vi "Wait for application to close.vi"(8 "error in (no error)":errorcluster, 11 "Applcation name":string="C:\\\\WINDOWS\\\\SYSTEM32\\\\cmd.exe") -> (0 "error out":errorcluster)   [LabVIEW 2013]
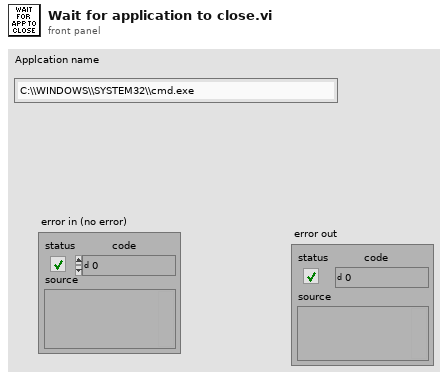
[diagram p1: front panel]
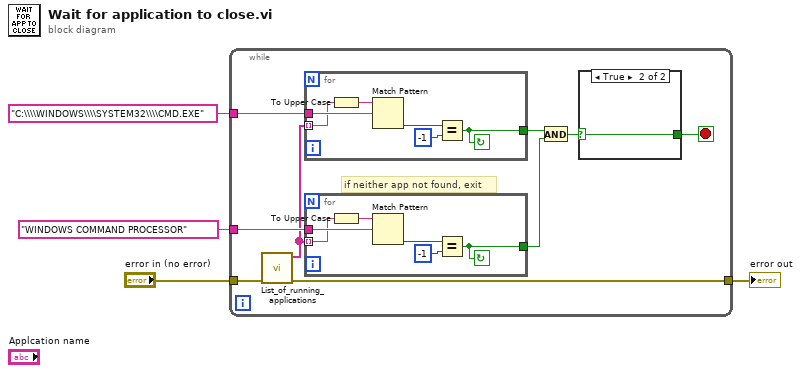
[diagram p0: block diagram]
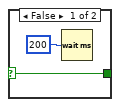
[diagram p2: hidden frame]
diagram:
  n1 = while {
    tunnel: "error in (no error)" -> [w12]
    tunnel: [w11] -> w3
    tunnel: "WINDOWS COMMAND PROCESSOR" -> [w10]
    tunnel: "C:\\\\WINDOWS\\\\SYSTEM32\\\\CMD.EXE" ("Applcation name") -> [w8]
    stop <- w13 stop-if-true
    # "if neither app not found, exit"
    n2 = call "List_of_running_applications.vi"("error in (no error)"=w12) -> ("error out"=w11:errorcluster, "TaskManager's list"=w9:string[])  [unwired: 7 in]
    n3 = for {
      tunnel: w9 -> [w15] mode=indexing
      tunnel: [w16] -> w7
      tunnel: w8 -> [w17]
      stop <- w16 continue-if-true
      n4 = To Upper Case(1:w15) -> (0:w14:string)
      n5 = Match Pattern(string=w14, regular expression=w17) -> (offset past match=w19:i32)  [unwired: 1 in, 3 out]
      n6 = Equal?(x=w19, y=-1) -> (x = y?=w16:bool)
    }
    n7 = for {
      tunnel: w9 -> [w24] mode=indexing
      tunnel: [w26] -> w6
      tunnel: w10 -> [w25]
      stop <- w26 continue-if-true
      n8 = To Upper Case(1:w24) -> (0:w23:string)
      n9 = Match Pattern(string=w23, regular expression=w25) -> (offset past match=w28:i32)  [unwired: 1 in, 3 out]
      n10 = Equal?(x=w28, y=-1) -> (x = y?=w26:bool)
    }
    n11 = And(x=w7, y=w6) -> (x .and. y?=w5:bool)
    n12 = case shown="True" w5 {
      selector: w5 -> [w20 w22]
      tunnel: [w20 w22] -> w13
      frame False {
        n13 = Wait (ms)(milliseconds to wait=u32 200) -> ()  [unwired: 1 out]
      }
      frame True {
      }
    }
  }
  "error out" <- w3
